vi "PatchViewer.vi"() -> ()   [LabVIEW 2014]
uses:
  <vilib>/Utility/sysdir.llb/System Directory Type.ctl
  <vilib>/Utility/file.llb/Read From Spreadsheet File (DBL).vi
  <vilib>/Utility/file.llb/Write To Spreadsheet File (DBL).vi
  <vilib>/vision/NI_Vision_Development_Module.lvlib
  <vilib>/ptbypt/NI_PtbyPt.lvlib
panel:
  in  "Diff":dbl
  in  "REC":bool
  out "all rows":dbl[][](array[numeric])
  in  "Gamma":dbl(slide)=0.5 min=0.5 max=2.0 step=0.1 scale=0.5..2.0
  in  "Contrast":i64(slide) caption="Gain (Raw)" min=0 max=384 step=1 scale=0.0..100.0
  in  "AutoContrast":bool
  in  "AutoExposure":bool
  in  "Decrease":bool
  in  "Increase":bool
  in  "set 4":bool
  in  "set 3":bool
  in  "set 2":bool
  in  "set 1":bool
  in  "pos 4":bool
  in  "pos 3":bool
  in  "pos 2":bool
  in  "pos 1":bool
  in  "zoom 4":bool
  in  "zoom 3":bool
  in  "zoom 2":bool
  in  "zoom1":bool
  out "fps":dbl
  in  "stop":bool
  in  "Gain":dbl(slide)=1.0 min=1.0 max=4.0 scale=1.0..4.0
  in  "Exposure Time (ms)":dbl(slide)=32000.0 caption="Exposure Time" min=2000.0 max=32000.0 scale=2000.0..32000.0 scale format="%^#_3g"
  out "Image Out":T1(plugin-control)
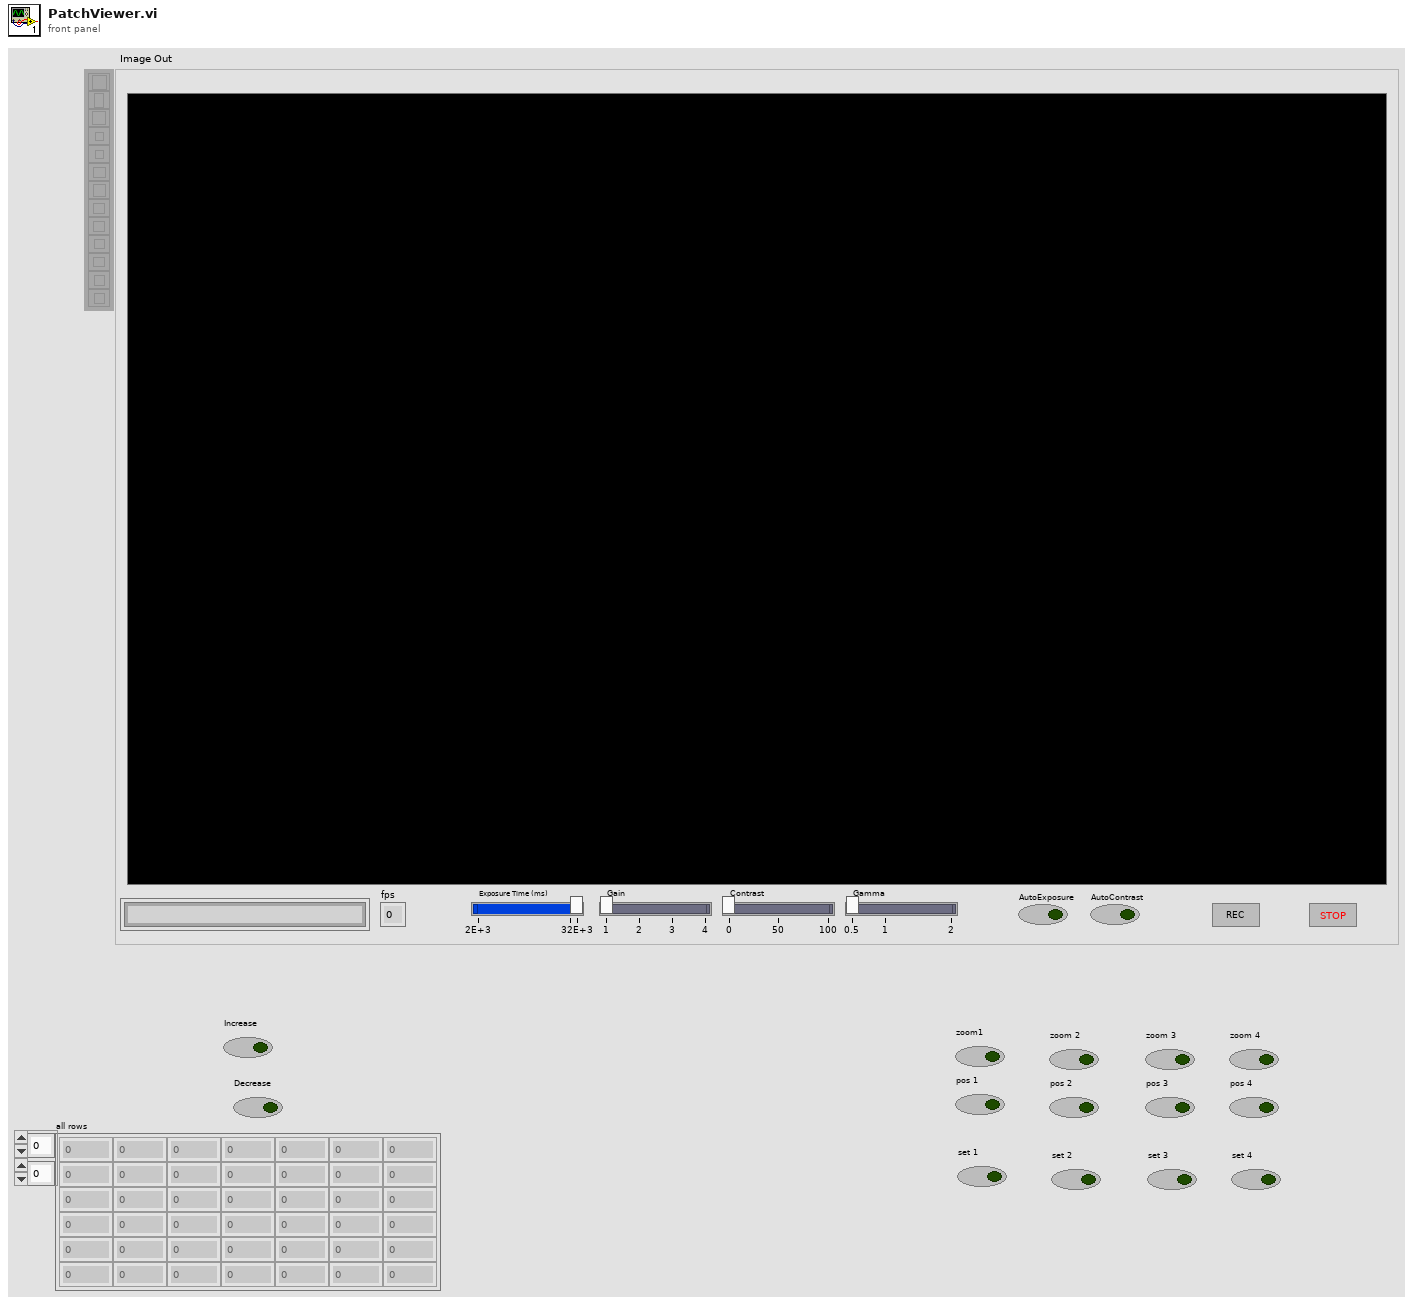
[diagram p1: front panel]
types:
  T1 = typedef "IMAQ Image.ctl" = refnum<image>
  T2 = cluster{"Brightness":sgl, "Contrast":sgl, "Gamma":sgl}
  T3 = cluster{"Mean Value":sgl, "Standard Variation":sgl, "Minimal Value":sgl, "Maximal Value":sgl, "Area (calibrated)":sgl, "Area (pixels)":u32, "%":sgl, "Calibration Valid":bool}
  T4 = typedef "System Directory Type.ctl" = i32
  T5 = typedef "IMAQ AVI2 Refnum.ctl" = refnum<k20>
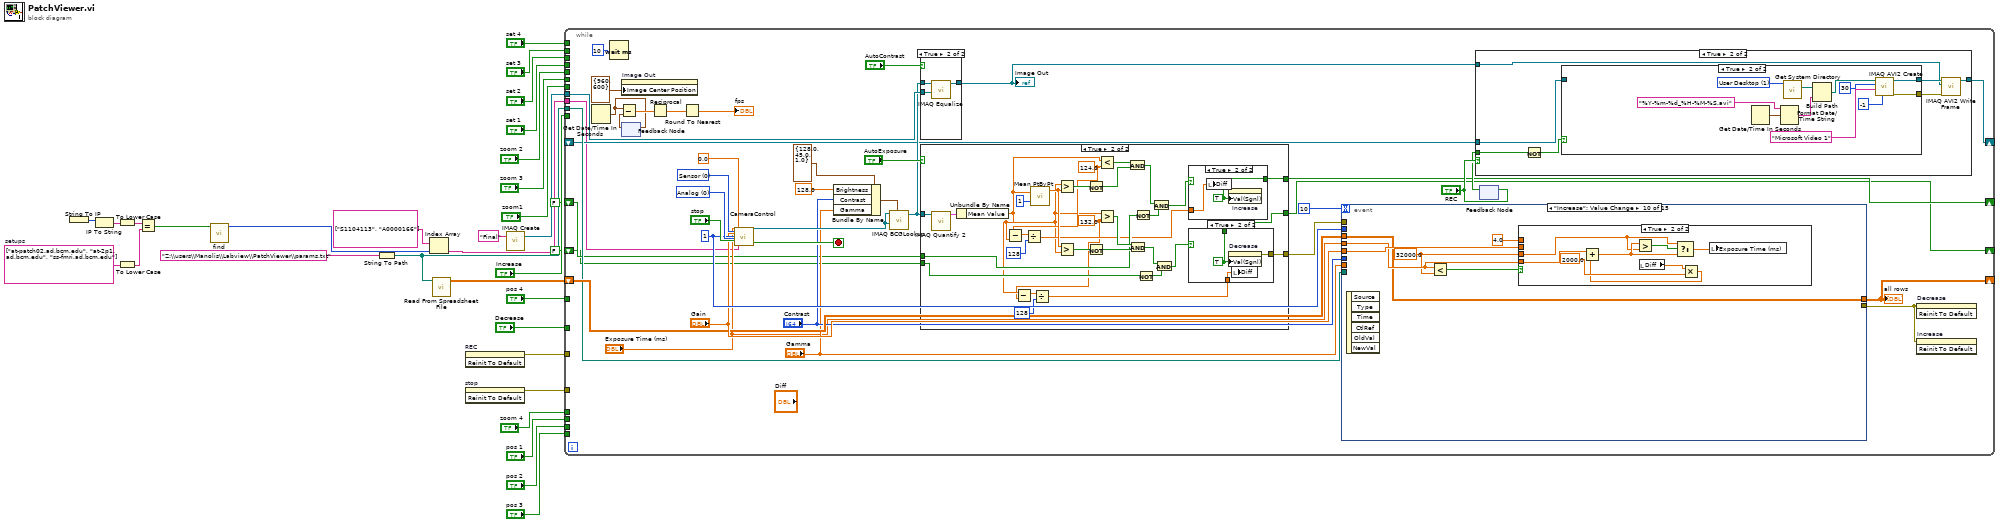
[diagram p0: block diagram]
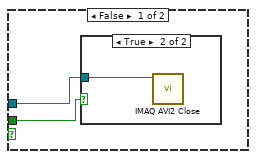
[diagram p2: hidden frame]
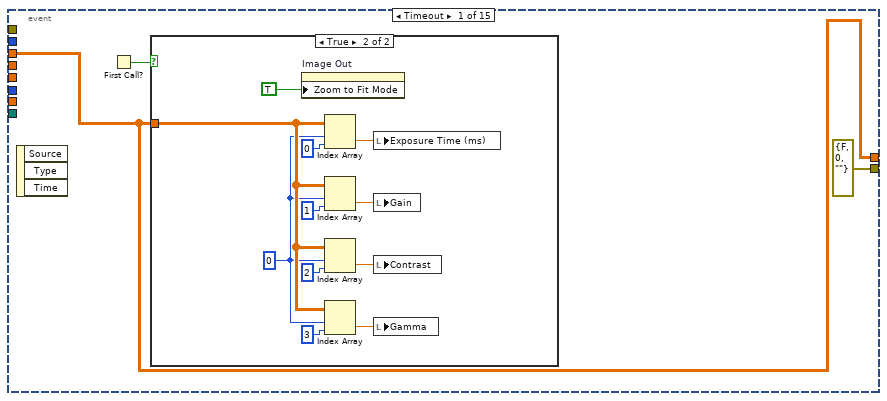
[diagram p9: hidden frame]
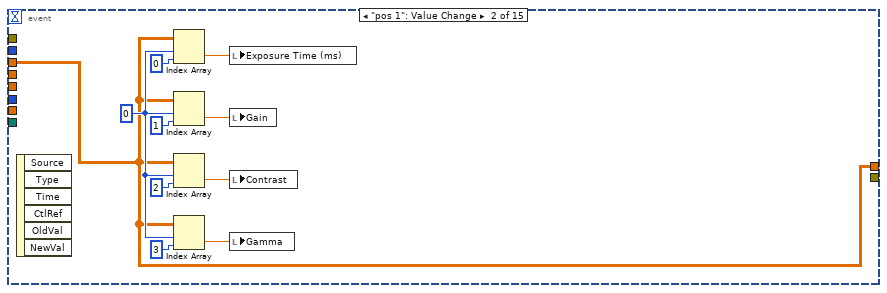
[diagram p11: hidden frame]
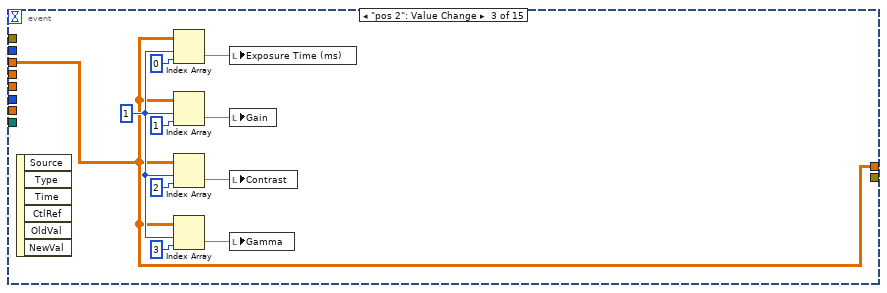
[diagram p12: hidden frame]
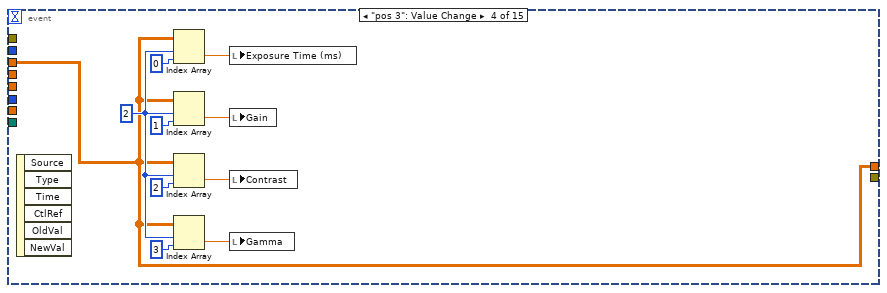
[diagram p13: hidden frame]
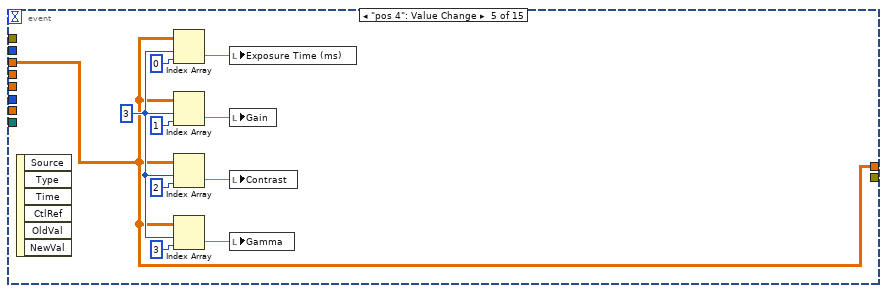
[diagram p14: hidden frame]
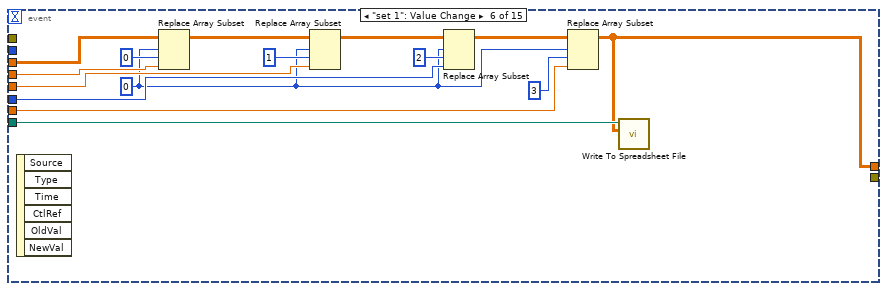
[diagram p15: hidden frame]
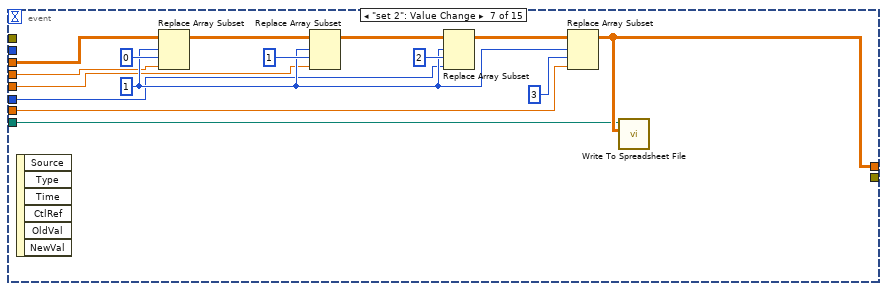
[diagram p16: hidden frame]
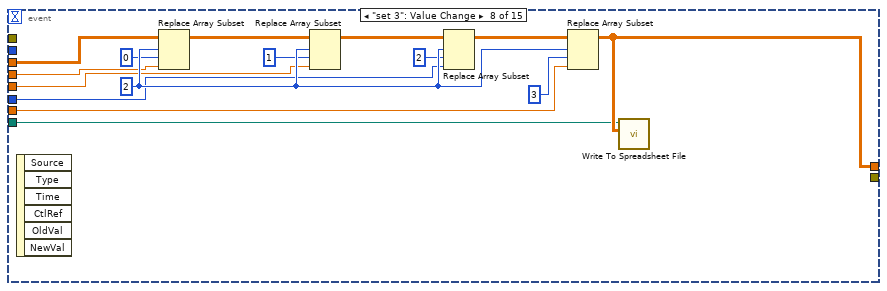
[diagram p17: hidden frame]
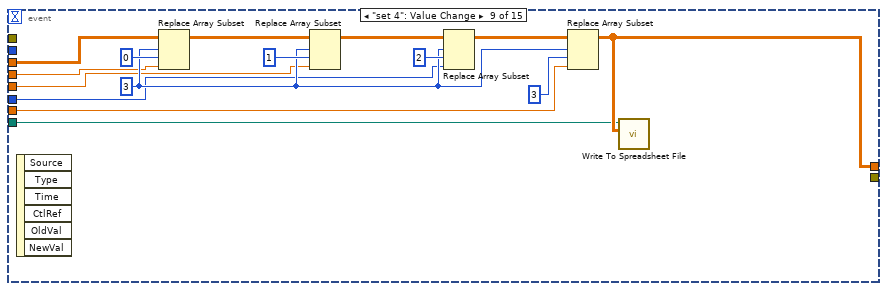
[diagram p18: hidden frame]
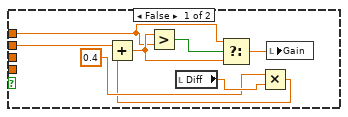
[diagram p19: hidden frame]
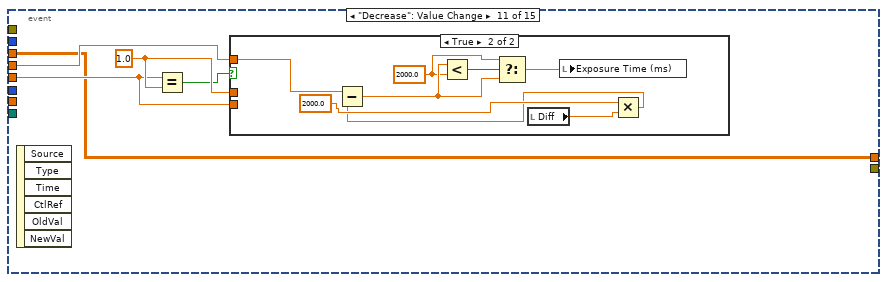
[diagram p20: hidden frame]
diagram:
  w8 = string[] ["at-patch02.ad.bcm.edu", "at-2p1.ad.bcm.edu", "ss-fmri.ad.bcm.edu"]  # setups
  n1 = String To IP() -> (0:w11:u32)  [unwired: 1 in]
  n2 = IP To String(2:w11) -> (0:w10:string)  [unwired: 1 in]
  n3 = To Lower Case(string=w10) -> (all lower case string=w9:string)
  n4 = To Lower Case(string=w8) -> (all lower case string=w7:string[])
  n5 = Equal?(x=w9, y=w7) -> (x = y?=w6:bool[])
  n6 = call "find.vi"("Array"=w6) -> ("Index"=w5:i32)  [unwired: 10 in]
  n7 = String To Path(string="Z:\\users\\Manolis\\Labview\\PatchViewer\\params.txt") -> (path=w14:path)
  n8 = Index Array(array=string[] ["S1104113", "A0000166"], index=w5) -> (element=w3:string)
  n9 = call-poly <vilib>:"Read From Spreadsheet File.vi"("file path (dialog if empty)"=w14) -> ("all rows"=w15:dbl[][])  [unwired: 6 in, 4 out]
  n10 = invoke on="REC" class="Bool (strict)" method="Reinit To Default"() -> (error out=w13:errorcluster)  [unwired: 3 in, 2 out]
  n11 = invoke on="stop" class="Bool" method="Reinit To Default"() -> (error out=w12:errorcluster)  [unwired: 3 in, 2 out]
  n12 = call "IMAQ Create"("Image Name"="Final") -> ("New Image"=w17:T1)  [unwired: 4 in, 1 out]
  n13 = while {
    tunnel: "pos 4" -> [_]
    tunnel: "pos 3" -> [_]
    tunnel: "pos 2" -> [_]
    tunnel: "pos 1" -> [_]
    tunnel: "zoom1" -> [_]
    tunnel: "zoom 4" -> [_]
    tunnel: "set 4" -> [_]
    tunnel: "set 3" -> [_]
    tunnel: "set 2" -> [_]
    tunnel: "set 1" -> [_]
    tunnel: "zoom 2" -> [_]
    tunnel: "zoom 3" -> [_]
    tunnel: "Increase" -> [_]
    tunnel: "Decrease" -> [_]
    tunnel: w17 -> [w56]
    shift-right: [w53] -> _
    shift-left: w15 -> [w54]
    tunnel: w14 -> [w52]
    shift-right: [w41] -> _
    shift-left: _ -> [w40]
    tunnel: w13 -> [_]
    tunnel: w12 -> [_]
    tunnel: w3 -> [w37]
    shift-right: [w36] -> _
    shift-left: FALSE ("Value (Signaling)") -> [w35]
    shift-right: [w34] -> _
    shift-left: FALSE ("Value (Signaling)") -> [w33]
    stop <- w73 stop-if-true
    w61 = i64 1 ("Gain (Raw)")
    w71 = u32 0 items=["Analog"] ("Black Level Selector")
    w72 = u32 0 items=["Sensor", "Digital"] ("Gain Selector")
    n14 = Get Date/Time In Seconds() -> (seconds since 1Jan1904=w67:timestamp)
    n15 = Wait (ms)(milliseconds to wait=u32 10) -> ()  [unwired: 1 out]
    n16 = property on="Image Out" class="ImageControl"("Image Center Position"=cluster{"X":u32, "Y":u32} {"X"=960, "Y"=600} ("Image Center Position:All Elements")) -> ()  [unwired: 2 in, 2 out]
    n17 = feedback-in #1(w67) -> ()
    n18 = feedback #1() -> (w66:timestamp)  [unwired: 1 in]
    n19 = Subtract(x=w67, y=w66) -> (x-y=w68:dbl)
    n20 = Reciprocal(x=w68) -> (1/x=w65:dbl)
    n21 = Round To Nearest(number=w65) -> (nearest integer value=→"fps":dbl)
    n22 = call "CameraControl.vi"("Exposure Time"="Exposure Time (ms)", "Gain Selector"=w72, "Gain"="Gain", "Gain (Raw)"=w61, "Black Level Selector"=w71, "Stop (F)"="stop", "Black Level"=0.0, "Camera"=w37) -> ("Image Out"=w51:T1, "Stopped"=w73:bool)  [unwired: 15 in, 3 out]
    n23 = Bundle By Name(cluster=T2 {"Brightness"=128.0, "Contrast"=45.0, "Gamma"=1.0} ("BCG Values"), "Brightness"=sgl 128.0, "Contrast"="Contrast", "Gamma"="Gamma") -> (w44:T2)
    n24 = call "IMAQ BCGLookup"("Image Src"=w51, "BCG Values"=w44, "Image Dst"=w51) -> ("Image Dst Out"=w49:T1)  [unwired: 4 in, 1 out]
    n25 = case shown="True" "AutoContrast" {
      tunnel: [w96 w98] -> w39
      tunnel: w49 -> [w96 w99]
      tunnel: w56 -> [_ w97]
      frame False {
      }
      frame True {
        n26 = call "IMAQ Equalize"("Image Dst"=w97, "Image Src"=w99) -> ("Image Dst Out"=w98:T1)  [unwired: 8 in, 1 out]
      }
    }
    "Image Out" <- w39
    n27 = case shown="True" "AutoExposure" {
      tunnel: w49 -> [_ w129]
      tunnel: [_ w128] -> w58
      tunnel: [_ w118] -> w36
      tunnel: w35 -> [_ w113]
      tunnel: [_ w117] -> w34
      tunnel: w33 -> [_ w109]
      frame False {
      }
      frame True {
        w108 = sgl 124.0 ("y")
        w101 = sgl 132.0 ("y")
        n28 = call "IMAQ Quantify 2"("Image"=w129) -> ("Global Report"=w119:T3)  [unwired: 8 in, 2 out]
        n29 = Unbundle By Name(w119) -> ("Mean Value"=w102:sgl)
        n30 = Subtract(x=w108, y=w102) -> (x-y=w106:sgl)
        n31 = Subtract(x=w102, y=w101) -> (x-y=w103:sgl)
        n32 = Divide(x=w106, y=128) -> (x/y=w105:sgl)
        n33 = call <vilib>:"Mean PtByPt.vi"("x"=w102, "sample length"=1) -> ("mean"=w121:dbl)  [unwired: 2 in, 1 out]
        n34 = Divide(x=w103, y=128) -> (x/y=w100:sgl)
        n35 = Greater?(x=w102, y=w121) -> (0:w125:bool)
        n36 = Greater?(x=w121, y=w102) -> (0:w122:bool)
        n37 = Not(x=w125) -> (.not. x?=w124:bool)
        n38 = Not(x=w122) -> (.not. x?=w123:bool)
        n39 = Less?(x=w102, y=w108) -> (x < y?=w127:bool)
        n40 = Greater?(x=w102, y=w101) -> (0:w120:bool)
        n41 = And(x=w127, y=w124) -> (x .and. y?=w115:bool)
        n42 = And(x=w120, y=w123) -> (x .and. y?=w110:bool)
        n43 = Not(x=w113) -> (.not. x?=w116:bool)
        n44 = Not(x=w109) -> (.not. x?=w112:bool)
        n45 = And(x=w115, y=w116) -> (x .and. y?=w114:bool)
        n46 = And(x=w110, y=w112) -> (x .and. y?=w111:bool)
        n47 = case shown="True" w114 {
          selector: w114 -> [w130 _]
          tunnel: [w130 w132] -> w118
          tunnel: w105 -> [_ w131]
          frame False {
          }
          frame True {
            w132 = TRUE ("Value (Signaling)")
            n48 = local write "Diff"(w131) -> ()
            n49 = property on="Increase" class="Bool (strict)"("Val(Sgnl)"=w132) -> ()  [unwired: 2 in, 2 out]
          }
        }
        n50 = case shown="True" w111 {
          selector: w111 -> [w133 _]
          tunnel: [_ w136] -> w128
          tunnel: [w133 w135] -> w117
          tunnel: w100 -> [_ w134]
          frame False {
          }
          frame True {
            w135 = TRUE ("Value (Signaling)")
            n51 = property on="Decrease" class="Bool (strict)"("Val(Sgnl)"=w135) -> (error out=w136:errorcluster)  [unwired: 2 in, 1 out]
            n52 = local write "Diff"(w134) -> ()
          }
        }
      }
    }
    n53 = event shown="[9] \"Increase\": Value Change" {
      selector: _ -> [_ _ _ _ _ _ _ _ _ _ _ _ _ _ _]
      dyn-events: _ -> [_ _ _ _ _ _ _ _ _ _ _ _ _ _ _]
      timeout: 10 -> [_ _ _ _ _ _ _ _ _ _ _ _ _ _ _]
      tunnel: "Exposure Time (ms)" -> [_ _ _ _ _ w205 w210 w224 w239 w254 w275 _ _ _ _]
      tunnel: w61 -> [_ _ _ _ _ _ _ _ _ _ _ _ _ _ _]
      tunnel: "Gain" -> [_ _ _ _ _ w204 w209 w223 w238 w256 w276 _ _ _ _]
      tunnel: "Contrast" -> [_ _ _ _ _ w202 w212 w226 w241 _ _ _ _ _ _]
      tunnel: "Gamma" -> [_ _ _ _ _ w201 w211 w225 w240 _ _ _ _ _ _]
      tunnel: [errorcluster {"status"=FALSE, "code"=0, "source"=""} ("error out") _ _ _ _ _ _ _ _ _ _ _ _ _ _] -> w59
      tunnel: w58 -> [_ _ _ _ _ _ _ _ _ _ _ _ _ _ _]
      tunnel: w54 -> [w137 w151 w161 w171 w181 w203 w208 w227 w242 w253 w274 w294 w298 w302 w307]
      tunnel: [w137 w151 w161 w171 w181 w191 w207 w222 w237 w253 w274 w294 w298 w302 w307] -> w53
      tunnel: w52 -> [_ _ _ _ _ w192 w206 w221 w236 _ _ _ _ _ _]
      event Timeout {
        n54 = event-data() -> ()  [unwired: 1 in, 3 out]
        n55 = First Call?() -> (First Call?: T/F=w138:bool)
        n56 = case shown="True" w138 {
          tunnel: w137 -> [_ w149]
          frame False {
          }
          frame True {
            w141 = 0 ("index (row)")
            n57 = property on="Image Out" class="ImageControl"("Zoom to Fit Mode"=TRUE) -> ()  [unwired: 2 in, 2 out]
            n58 = Index Array(array=w149, index (row)=w141, index (col)=0 ("disabled index (col)")) -> (element=w145:dbl)
            n59 = Index Array(array=w149, index (row)=w141, index (col)=1 ("disabled index (col)")) -> (element=w144:dbl)
            n60 = Index Array(array=w149, index (row)=w141, index (col)=2 ("disabled index (col)")) -> (element=w143:dbl)
            n61 = Index Array(array=w149, index (row)=w141, index (col)=3 ("disabled index (col)")) -> (element=w142:dbl)
            n62 = local write "Exposure Time (ms)"(w145) -> ()
            n63 = local write "Gain"(w144) -> ()
            n64 = local write "Contrast"(w143) -> ()
            n65 = local write "Gamma"(w142) -> ()
          }
        }
      }
      event "pos 1": Value Change {
        w160 = 0 ("index (row)")
        n66 = event-data() -> ()  [unwired: 1 in, 6 out]
        n67 = Index Array(array=w151, index (row)=w160, index (col)=0 ("disabled index (col)")) -> (element=w156:dbl)
        n68 = Index Array(array=w151, index (row)=w160, index (col)=1 ("disabled index (col)")) -> (element=w157:dbl)
        n69 = Index Array(array=w151, index (row)=w160, index (col)=2 ("disabled index (col)")) -> (element=w158:dbl)
        n70 = Index Array(array=w151, index (row)=w160, index (col)=3 ("disabled index (col)")) -> (element=w159:dbl)
        n71 = local write "Exposure Time (ms)"(w156) -> ()
        n72 = local write "Gain"(w157) -> ()
        n73 = local write "Contrast"(w158) -> ()
        n74 = local write "Gamma"(w159) -> ()
      }
      event "pos 2": Value Change {
        w162 = 1 ("index (row)")
        n75 = event-data() -> ()  [unwired: 1 in, 6 out]
        n76 = Index Array(array=w161, index (row)=w162, index (col)=0 ("disabled index (col)")) -> (element=w166:dbl)
        n77 = Index Array(array=w161, index (row)=w162, index (col)=1 ("disabled index (col)")) -> (element=w165:dbl)
        n78 = Index Array(array=w161, index (row)=w162, index (col)=2 ("disabled index (col)")) -> (element=w164:dbl)
        n79 = Index Array(array=w161, index (row)=w162, index (col)=3 ("disabled index (col)")) -> (element=w163:dbl)
        n80 = local write "Exposure Time (ms)"(w166) -> ()
        n81 = local write "Gain"(w165) -> ()
        n82 = local write "Contrast"(w164) -> ()
        n83 = local write "Gamma"(w163) -> ()
      }
      event "pos 3": Value Change {
        w180 = 2 ("index (row)")
        n84 = event-data() -> ()  [unwired: 1 in, 6 out]
        n85 = Index Array(array=w171, index (row)=w180, index (col)=0 ("disabled index (col)")) -> (element=w176:dbl)
        n86 = Index Array(array=w171, index (row)=w180, index (col)=1 ("disabled index (col)")) -> (element=w177:dbl)
        n87 = Index Array(array=w171, index (row)=w180, index (col)=2 ("disabled index (col)")) -> (element=w178:dbl)
        n88 = Index Array(array=w171, index (row)=w180, index (col)=3 ("disabled index (col)")) -> (element=w179:dbl)
        n89 = local write "Exposure Time (ms)"(w176) -> ()
        n90 = local write "Gain"(w177) -> ()
        n91 = local write "Contrast"(w178) -> ()
        n92 = local write "Gamma"(w179) -> ()
      }
      event "pos 4": Value Change {
        w182 = 3 ("index (row)")
        n93 = event-data() -> ()  [unwired: 1 in, 6 out]
        n94 = Index Array(array=w181, index (row)=w182, index (col)=0 ("disabled index (col)")) -> (element=w186:dbl)
        n95 = Index Array(array=w181, index (row)=w182, index (col)=1 ("disabled index (col)")) -> (element=w185:dbl)
        n96 = Index Array(array=w181, index (row)=w182, index (col)=2 ("disabled index (col)")) -> (element=w184:dbl)
        n97 = Index Array(array=w181, index (row)=w182, index (col)=3 ("disabled index (col)")) -> (element=w183:dbl)
        n98 = local write "Exposure Time (ms)"(w186) -> ()
        n99 = local write "Gain"(w185) -> ()
        n100 = local write "Contrast"(w184) -> ()
        n101 = local write "Gamma"(w183) -> ()
      }
      event "set 1": Value Change {
        w193 = 0 ("index (row)")
        n102 = event-data() -> ()  [unwired: 1 in, 6 out]
        n103 = Replace Array Subset(array=w203, new element=w205, index (row)=w193, index (col)=0 ("index (row)")) -> (w200:dbl[][])
        n104 = Replace Array Subset(array=w200, new element=w204, index (row)=w193, index (col)=1 ("index (row)")) -> (w199:dbl[][])
        n105 = Replace Array Subset(array=w199, new element=w202, index (row)=w193, index (col)=2 ("index (row)")) -> (w198:dbl[][])
        n106 = Replace Array Subset(array=w198, new element=w201, index (row)=w193, index (col)=3 ("index (row)")) -> (w191:dbl[][])
        n107 = call-poly <vilib>:"Write To Spreadsheet File.vi"("2D data"=w191, "file path (dialog if empty)"=w192) -> ()  [unwired: 6 in, 1 out]
      }
      event "set 2": Value Change {
        w213 = 1 ("index (row)")
        n108 = event-data() -> ()  [unwired: 1 in, 6 out]
        n109 = Replace Array Subset(array=w208, new element=w210, index (row)=w213, index (col)=0 ("index (row)")) -> (w220:dbl[][])
        n110 = Replace Array Subset(array=w220, new element=w209, index (row)=w213, index (col)=1 ("index (row)")) -> (w219:dbl[][])
        n111 = Replace Array Subset(array=w219, new element=w212, index (row)=w213, index (col)=2 ("index (row)")) -> (w218:dbl[][])
        n112 = Replace Array Subset(array=w218, new element=w211, index (row)=w213, index (col)=3 ("index (row)")) -> (w207:dbl[][])
        n113 = call-poly <vilib>:"Write To Spreadsheet File.vi"("2D data"=w207, "file path (dialog if empty)"=w206) -> ()  [unwired: 6 in, 1 out]
      }
      event "set 3": Value Change {
        w235 = 2 ("index (row)")
        n114 = event-data() -> ()  [unwired: 1 in, 6 out]
        n115 = Replace Array Subset(array=w227, new element=w224, index (row)=w235, index (col)=0 ("index (row)")) -> (w228:dbl[][])
        n116 = Replace Array Subset(array=w228, new element=w223, index (row)=w235, index (col)=1 ("index (row)")) -> (w229:dbl[][])
        n117 = Replace Array Subset(array=w229, new element=w226, index (row)=w235, index (col)=2 ("index (row)")) -> (w230:dbl[][])
        n118 = Replace Array Subset(array=w230, new element=w225, index (row)=w235, index (col)=3 ("index (row)")) -> (w222:dbl[][])
        n119 = call-poly <vilib>:"Write To Spreadsheet File.vi"("2D data"=w222, "file path (dialog if empty)"=w221) -> ()  [unwired: 6 in, 1 out]
      }
      event "set 4": Value Change {
        w243 = 3 ("index (row)")
        n120 = event-data() -> ()  [unwired: 1 in, 6 out]
        n121 = Replace Array Subset(array=w242, new element=w239, index (row)=w243, index (col)=0 ("index (row)")) -> (w250:dbl[][])
        n122 = Replace Array Subset(array=w250, new element=w238, index (row)=w243, index (col)=1 ("index (row)")) -> (w249:dbl[][])
        n123 = Replace Array Subset(array=w249, new element=w241, index (row)=w243, index (col)=2 ("index (row)")) -> (w248:dbl[][])
        n124 = Replace Array Subset(array=w248, new element=w240, index (row)=w243, index (col)=3 ("index (row)")) -> (w237:dbl[][])
        n125 = call-poly <vilib>:"Write To Spreadsheet File.vi"("2D data"=w237, "file path (dialog if empty)"=w236) -> ()  [unwired: 6 in, 1 out]
      }
      event "Increase": Value Change {
        w251 = 32000.0 ("y")
        n126 = event-data() -> ()  [unwired: 1 in, 6 out]
        n127 = Less?(x=w254, y=w251) -> (x < y?=w252:bool)
        n128 = case shown="True" w252 {
          tunnel: w254 -> [_ w272]
          tunnel: w256 -> [w264 _]
          tunnel: 4.0 ("y") -> [w260 _]
          tunnel: w251 -> [_ w268]
          frame False {
            n129 = local read "Diff"() -> (w259:dbl)
            n130 = Multiply(x=0.4 ("y"), y=w259) -> (x*y=w257:dbl)
            n131 = Add(x=w264, y=w257) -> (x+y=w262:dbl)
            n132 = Greater?(x=w262, y=w260) -> (0:w263:bool)
            n133 = Select(t=w260, s=w263, f=w262) -> (s? t:f=w261:dbl)
            n134 = local write "Gain"(w261) -> ()
          }
          frame True {
            n135 = local read "Diff"() -> (w267:dbl)
            n136 = Multiply(x=w267, y=2000.0) -> (x*y=w265:dbl)
            n137 = Add(x=w272, y=w265) -> (x+y=w270:dbl)
            n138 = Greater?(x=w270, y=w268) -> (0:w271:bool)
            n139 = Select(t=w268, s=w271, f=w270) -> (s? t:f=w269:dbl)
            n140 = local write "Exposure Time (ms)"(w269) -> ()
          }
        }
      }
      event "Decrease": Value Change {
        w277 = 1.0 ("y")
        n141 = event-data() -> ()  [unwired: 1 in, 6 out]
        n142 = Equal?(x=w276, y=w277) -> (x = y?=w273:bool)
        n143 = case shown="True" w273 {
          tunnel: w275 -> [_ w293]
          tunnel: w276 -> [w285 _]
          tunnel: w277 -> [w281 _]
          frame False {
            n144 = local read "Diff"() -> (w280:dbl)
            n145 = Multiply(x=0.4 ("y"), y=w280) -> (x*y=w278:dbl)
            n146 = Subtract(x=w285, y=w278) -> (x-y=w283:dbl)
            n147 = Less?(x=w283, y=w281) -> (x < y?=w284:bool)
            n148 = Select(t=w281, s=w284, f=w283) -> (s? t:f=w282:dbl)
            n149 = local write "Gain"(w282) -> ()
          }
          frame True {
            w290 = 2000.0 ("y")
            n150 = local read "Diff"() -> (w288:dbl)
            n151 = Multiply(x=2000.0 ("y"), y=w288) -> (x*y=w286:dbl)
            n152 = Subtract(x=w293, y=w286) -> (x-y=w291:dbl)
            n153 = Less?(x=w291, y=w290) -> (x < y?=w292:bool)
            n154 = Select(t=w290, s=w292, f=w291) -> (s? t:f=w289:dbl)
            n155 = local write "Exposure Time (ms)"(w289) -> ()
          }
        }
      }
      event "zoom1": Value Change {
        n156 = event-data() -> ()  [unwired: 1 in, 6 out]
        n157 = property on="Image Out" class="ImageControl"("Zoom to Fit Mode"=TRUE) -> ()  [unwired: 2 in, 2 out]
      }
      event "zoom 2": Value Change {
        w296 = 0.75
        n158 = event-data() -> ()  [unwired: 1 in, 6 out]
        n159 = Bundle By Name(cluster=cluster{"X":sgl, "Y":sgl} {"X"=0.0, "Y"=0.0} ("ZoomSingle:All Elements"), "X"=w296, "Y"=w296) -> (w299:cluster{"X":sgl, "Y":sgl})
        n160 = property on="Image Out" class="ImageControl"("ZoomSingle"=w299) -> ()  [unwired: 2 in, 2 out]
      }
      event "zoom 3": Value Change {
        w300 = 1.0
        n161 = event-data() -> ()  [unwired: 1 in, 6 out]
        n162 = Bundle By Name(cluster=cluster{"X":sgl, "Y":sgl} {"X"=0.0, "Y"=0.0} ("ZoomSingle:All Elements"), "X"=w300, "Y"=w300) -> (w303:cluster{"X":sgl, "Y":sgl})
        n163 = flat-sequence {
          tunnel: w303 -> [w304]
          frame #0 {
            n164 = property on="Image Out" class="ImageControl"("ZoomSingle"=w304) -> ()  [unwired: 2 in, 2 out]
          }
        }
      }
      event "zoom 4": Value Change {
        w305 = 1.5
        n165 = event-data() -> ()  [unwired: 1 in, 6 out]
        n166 = Bundle By Name(cluster=cluster{"X":sgl, "Y":sgl} {"X"=0.0, "Y"=0.0} ("ZoomSingle:All Elements"), "X"=w305, "Y"=w305) -> (w308:cluster{"X":sgl, "Y":sgl})
        n167 = flat-sequence {
          tunnel: w308 -> [w309]
          frame #0 {
            n168 = property on="Image Out" class="ImageControl"("ZoomSingle"=w309) -> ()  [unwired: 2 in, 2 out]
          }
        }
      }
    }
    "all rows" <- w53
    n169 = feedback #2() -> (w42:bool)  [unwired: 1 in]
    n170 = case shown="True" "REC" {
      tunnel: w39 -> [_ w81]
      tunnel: [_ w80] -> w41
      tunnel: w40 -> [w75 w79]
      tunnel: w42 -> [w74 w77]
      frame False {
        n171 = case shown="True" w74 {
          tunnel: w75 -> [_ w76]
          frame False {
          }
          frame True {
            n172 = call "IMAQ AVI2 Close"("AVI Refnum"=w76) -> ()  [unwired: 10 in, 1 out]
          }
        }
      }
      frame True {
        n173 = Not(x=w77) -> (.not. x?=w78:bool)
        n174 = case shown="True" w78 {
          tunnel: [w84 w95] -> w83
          tunnel: [_ w91] -> w82
          tunnel: w79 -> [w84 _]
          frame False {
          }
          frame True {
            w86 = T4 1 items=["User Home"=0, "User Desktop"=1, "User Documents"=2, "User Application Data"=3, "User Preferences"=4, "User Temporary"=5, "Public Documents"=6, "Public Application Data"=7, "Public Preferences"=8, "Public Cache"=13, "System Core Libraries"=9, "System Installed Libraries"=10, "Application Files"=11, "Boot Volume Root"=12] ("system directory type")
            n175 = Get Date/Time In Seconds() -> (seconds since 1Jan1904=w89:timestamp)
            n176 = Format Date/Time String(time format string (%c)="%Y-%m-%d_%H-%M-%S.avi", seconds (now)=w89) -> (date/time string=w90:string)  [unwired: 1 out]
            n177 = call <vilib>:"Get System Directory.vi"("system directory type"=w86) -> ("system directory"=w85:path)  [unwired: 10 in]
            n178 = Build Path(base path=w85, name or relative path=w90) -> (appended path=w87:path)
            n179 = call "IMAQ AVI2 Create"("Quality"=-1, "Codec"="Microsoft Video 1", "Frames Per Second"=u32 30, "AVI Path"=w87) -> ("error out"=w91:errorcluster, "AVI Refnum"=w95:T5)  [unwired: 6 in]
          }
        }
        n180 = call "IMAQ AVI2 Write Frame"("error in (no error)"=w82, "Image"=w81, "AVI Refnum"=w83) -> ("AVI Refnum (duplicate)"=w80:T5)  [unwired: 6 in, 2 out]
      }
    }
    n181 = feedback-in #2("REC") -> ()
    n182 = invoke on="Decrease" class="Bool (strict)" method="Reinit To Default"(error in=w59) -> ()  [unwired: 2 in, 3 out]
    n183 = invoke on="Increase" class="Bool (strict)" method="Reinit To Default"(error in=w59) -> ()  [unwired: 2 in, 3 out]
  }
